vi "Hilight Border Logic.vi"(10 "Hilight":bool, 11 "index":i32) -> (3 "Hilight":bool)   [LabVIEW 2025]
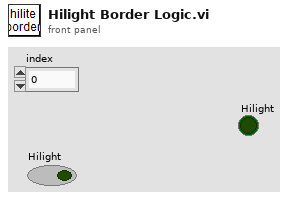
[diagram p1: front panel]
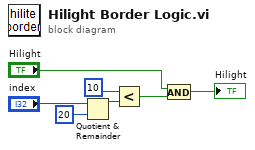
[diagram p0: block diagram]
diagram:
  n1 = Quotient & Remainder(x="index", y=20) -> (x-y*floor(x/y)=w4:i32)  [unwired: 1 out]
  n2 = Less?(x=10 ("y"), y=w4) -> (x < y?=w1:bool)
  n3 = And(x="Hilight", y=w1) -> (x .and. y?=→"Hilight":bool)
